vi "WriteReadDrag_YCC.vi"() -> ()   [LabVIEW 2014]
uses:
  (Global) Current handle and LaserPower_YCC.vi
panel:
  in  "Move to Position":bool
  in  "Clear one          all":bool
  in  "Clear Save Position":bool
  in  "Save Position":bool
  in  "Tab Control":enum32{"StandBy", "Drag", "Single WriteRead"}(tab)
  in  "Update new ADC(read) rate":bool
  out "Save Position (um)":dbl[][](array[numeric])
  in  "Clear index (row)":i32
  in  "Move index (row)":i32
  in  "Tab Control":T1(tab)
  in  "ADC Rate for 20bit (ms)":T2(ring)
  out "Sampling Rate for reading (Hz)":dbl
  in  "DAC rate (ms)":dbl=5.0
  out "DAC rate (Hz)":dbl
  out "XY Position":cluster{"X":dbl, "Y":dbl}[](graph)
  in  "Z  (um)":dbl=50.0 format="%.4f"
  out "Current Z (um)":dbl
  in  "Move Z?":bool
  in  "Adjust to Single Read":bool
  in  "Chang X?":bool
  in  "X Move to (um)":dbl=50.0 format="%_6g"
  in  "Chang Y?":bool
  in  "Y Move to (um)":dbl=50.0 format="%_6g"
  in  "Z Move to (um)":dbl=50.0 format="%_6g"
  in  "Chang Z?":bool
  in  "milliseconds to wait":u32=200
  out "Current Position Z (um)":dbl format="%.4f"
  out "Current Position Y (um)":dbl format="%.4f"
  out "Current Position X (um)":dbl format="%.4f"
  in  "read #":i32=1
  in  "Adjust to cursor":bool=TRUE
  in  "Move to (50,50,50) ?":bool
  in  "STOP":bool
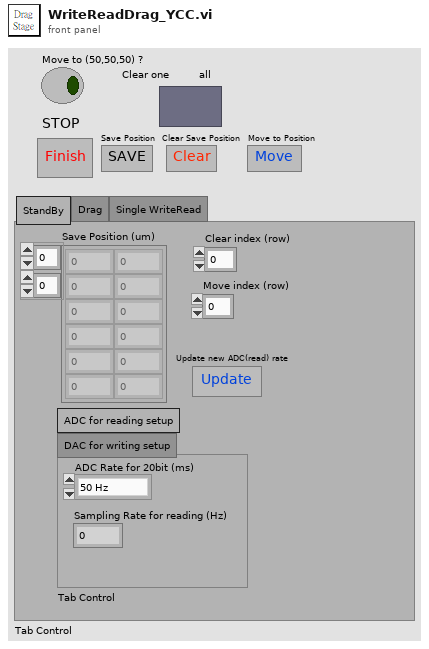
[diagram p1: front panel]
types:
  T1 = enum32{"ADC for reading setup", "DAC for writing setup"}
  T2 = enum16{"50 Hz", "60 Hz", "100 Hz", "500 Hz", "1000 Hz", "2000 Hz", "3750 Hz"}
  T3 = enum16{"StandBy", "Drag", "Single WriteRead", "Move to 50,50,50"}
  T4 = cluster{"Real Current Commanded position (um)":dbl, "Real Current Commanded position (um)":dbl}
  T5 = typedef "LVPointDoubleTypeDef.ctl" = cluster{"Cursor X":dbl, "Cursor Y":dbl}
  T6 = cluster{"position (um)":dbl, "position (um)":dbl}
  T7 = cluster{"Position wrote to three axis (um)":dbl, "Position wrote to three axis (um)":dbl}
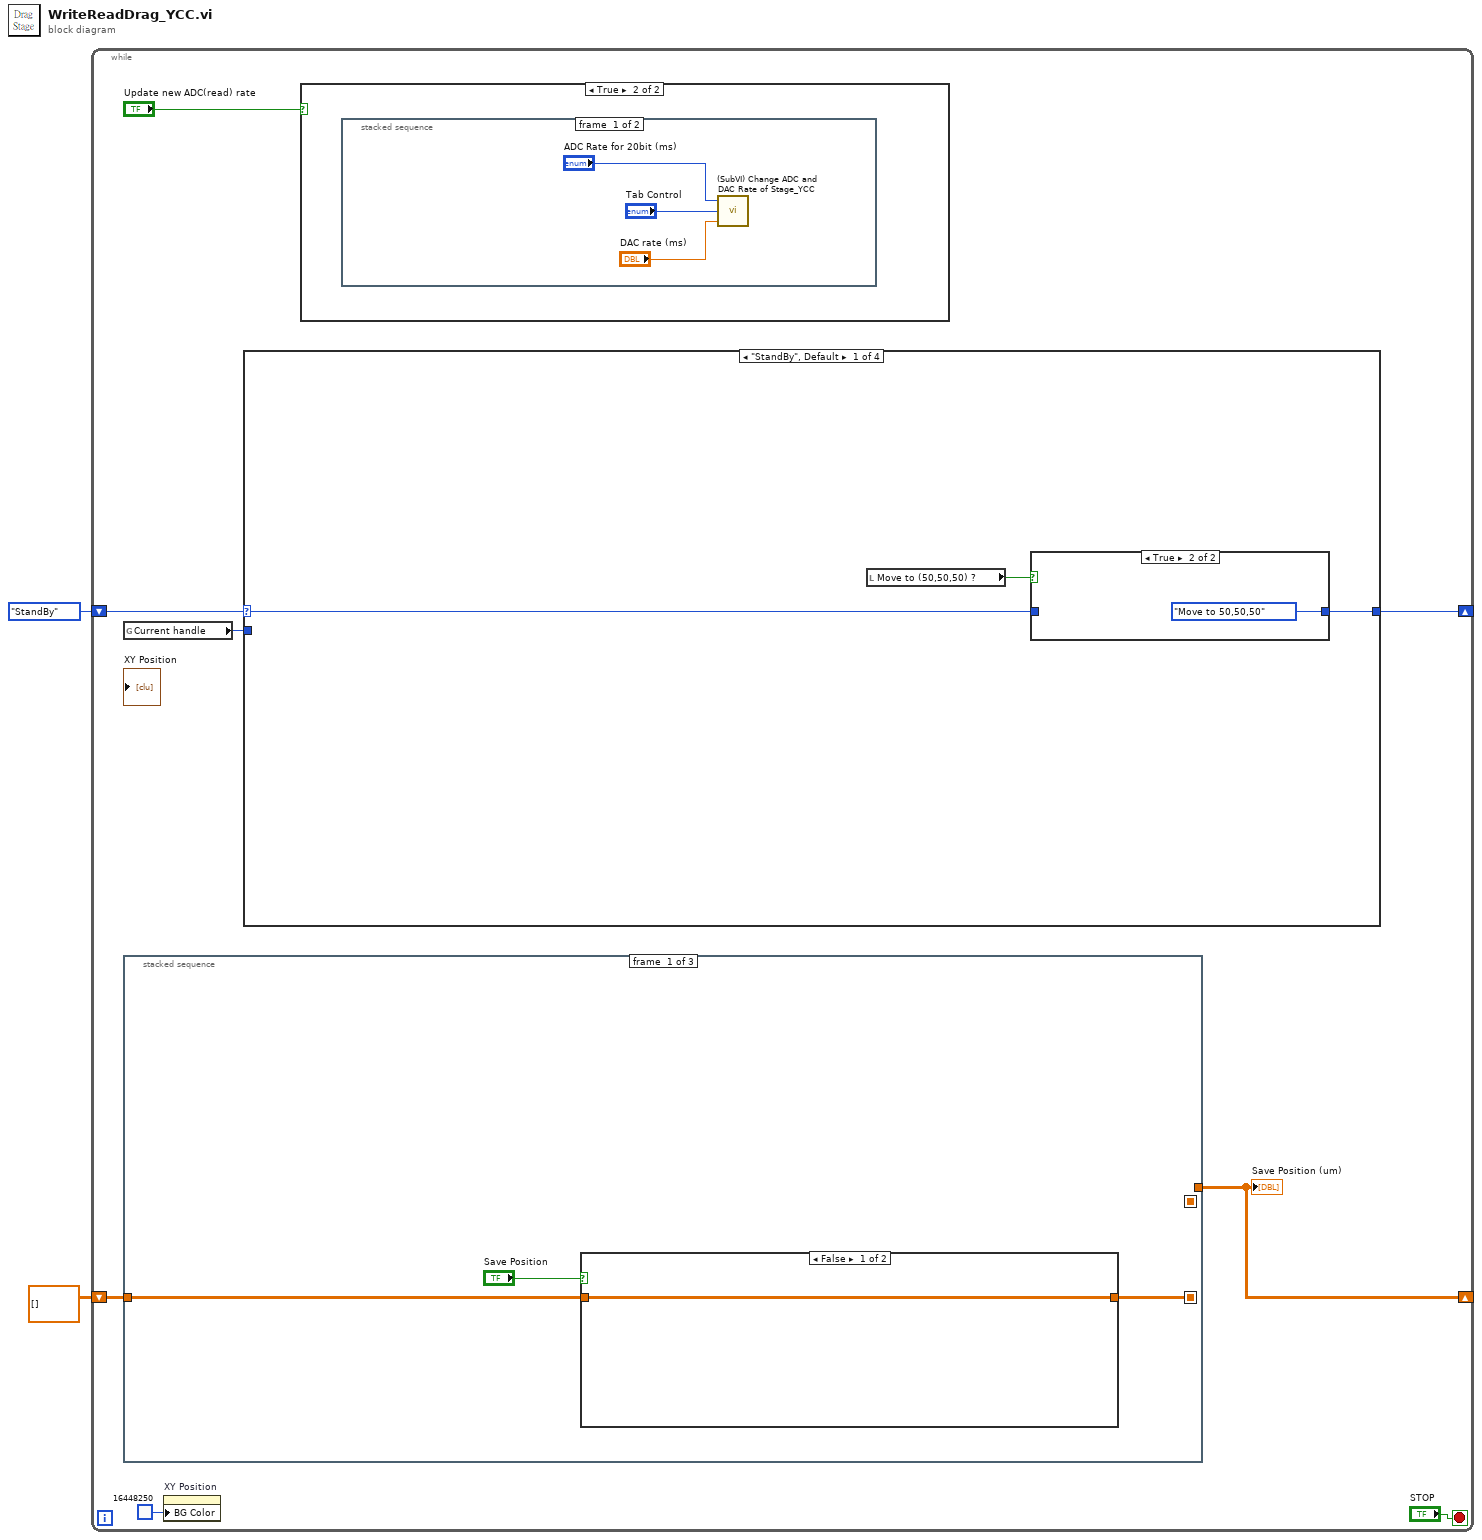
[diagram p0: block diagram]
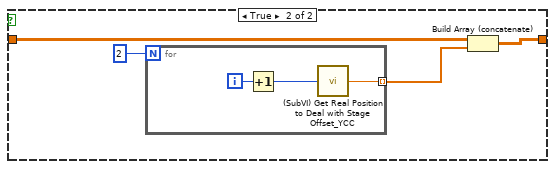
[diagram p2: hidden frame]
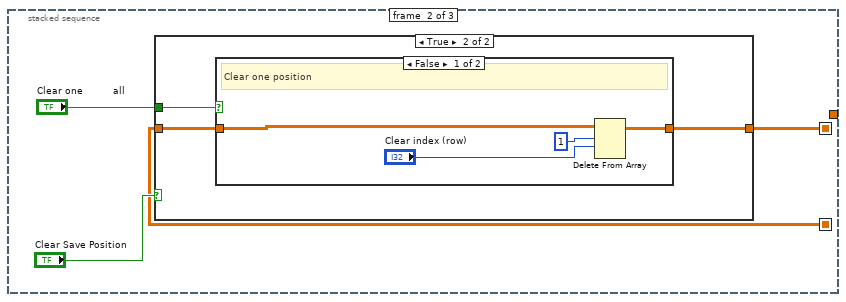
[diagram p3: hidden frame]
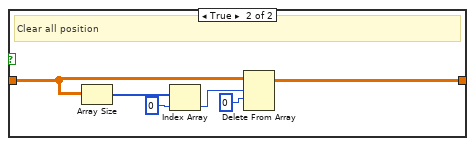
[diagram p5: hidden frame]
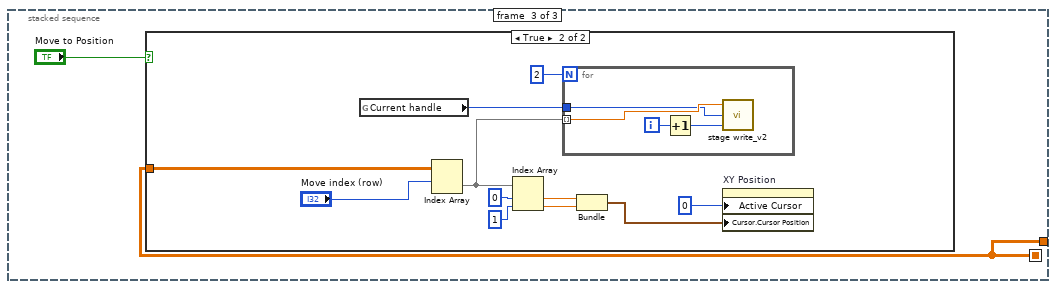
[diagram p6: hidden frame]
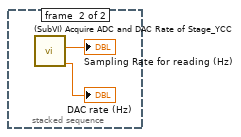
[diagram p9: hidden frame]
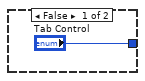
[diagram p10: hidden frame]
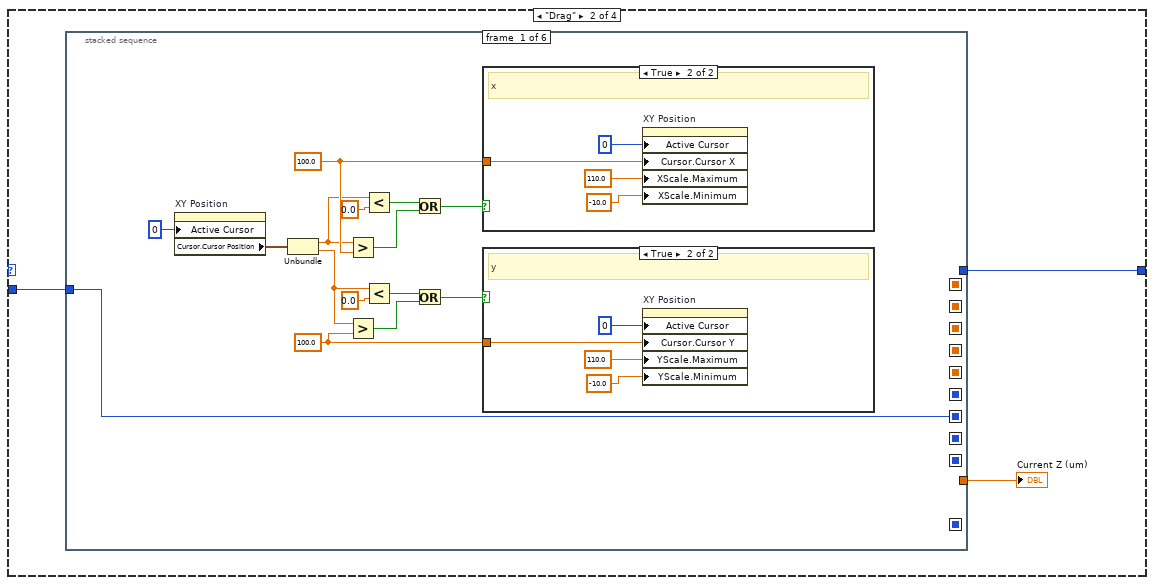
[diagram p11: hidden frame]
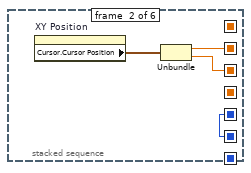
[diagram p14: hidden frame]
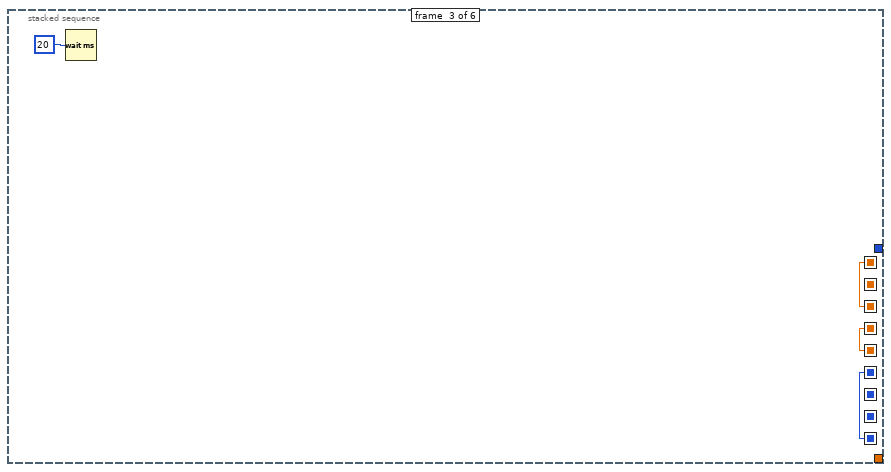
[diagram p15: hidden frame]
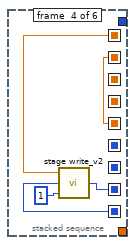
[diagram p16: hidden frame]
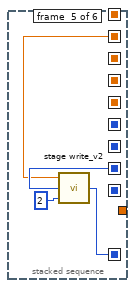
[diagram p17: hidden frame]
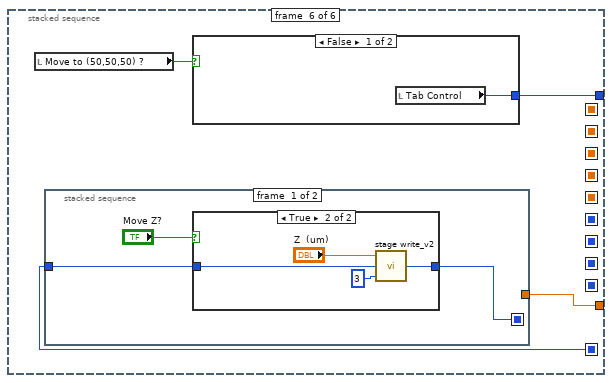
[diagram p18: hidden frame]
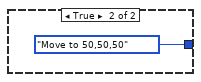
[diagram p19: hidden frame]
diagram:
  n1 = while {
    shift-right: [w10] -> _
    shift-left: T3."StandBy" ("Enum") -> [w8]
    shift-right: [w5] -> _
    shift-left: dbl[][] [] -> [w6]
    stop <- "STOP" stop-if-true
    n2 = global read "(Global) Current handle and LaserPower_YCC.vi" "Current handle"() -> (w7:i32)
    n3 = stacked-sequence {
      seq-local: [w11 _ _] -> [_ w23 _]
      seq-local: [_ w24 _] -> [_ _ w41]
      tunnel: w6 -> [w12 _ _]
      tunnel: [_ _ w41] -> w5
      frame #0 {
        n4 = case shown="False" "Save Position" {
          tunnel: [w14 w16] -> w11
          tunnel: w12 -> [w14 w15]
          frame False {
          }
          frame True {
            n5 = for {
              N: 2 -> [_]
              tunnel: [w19] -> w17 mode=indexing
              i -> [w21]
              n6 = Increment(x=w21) -> (x+1=w20:i32)
              n7 = call "(SubVI) Get Real Position to Deal with Stage Offset_YCC.vi"("Axis"=w20) -> ("Real Current Commanded position (um)"=w19:dbl)  [unwired: 3 in, 1 out]
            }
            n8 = Build Array (concatenate)(w15, w17) -> (w16:dbl[][])
          }
        }
      }
      frame #1 {
        n9 = case shown="True" "Clear Save Position" {
          tunnel: [w26 w27] -> w24
          tunnel: w23 -> [w26 w28]
          tunnel: "Clear one          all" -> [_ w29]
          frame False {
          }
          frame True {
            n10 = case shown="False" w29 {
              tunnel: w28 -> [w33 w39]
              tunnel: [w31 w34] -> w27
              frame False {
                # "Clear one position"
                n11 = Delete From Array(array=w33, length=1, index (row)="Clear index (row)") -> (array with subset deleted=w31:dbl[][])  [unwired: 1 in, 1 out]
              }
              frame True {
                # "Clear all position"
                n12 = Array Size(array=w39) -> (size(s)=w38:i32[])
                n13 = Index Array(array=w38, index=0) -> (element=w36:i32)
                n14 = Delete From Array(array=w39, length=w36, index (row)=0) -> (array with subset deleted=w34:dbl[][])  [unwired: 1 in, 1 out]
              }
            }
          }
        }
      }
      frame #2 {
        n15 = case shown="True" "Move to Position" {
          tunnel: w41 -> [_ w52]
          frame False {
          }
          frame True {
            n16 = global read "(Global) Current handle and LaserPower_YCC.vi" "Current handle"() -> (w49:i32)
            n17 = Index Array(array=w52, index (row)="Move index (row)") -> (element=w47:dbl[])  [unwired: 1 in]
            n18 = Index Array(array=w47, index #1=0 ("index"), index #2=1 ("index")) -> (element #1=w44:dbl, element #2=w43:dbl)
            n19 = for {
              N: 2 -> [_]
              tunnel: w47 -> [w56] mode=indexing
              tunnel: w49 -> [w53]
              i -> [w55]
              n20 = Increment(x=w55) -> (x+1=w54:i32)
              n21 = call "stage write_v2.vi"("axis"=w54, "Incoming Handle"=w53, "position"=w56) -> ()  [unwired: 2 in, 1 out]
            }
            n22 = Bundle("Real Current Commanded position (um)"=w44, "Real Current Commanded position (um)"=w43) -> (w42:T4)  [unwired: 1 in]
            n23 = property on="XY Position" class="XYGraph (strict)"("Active Cursor"=u32 0, "Cursor.Cursor Position"=w42) -> ()  [unwired: 2 in, 2 out]
          }
        }
      }
    }
    "Save Position (um)" <- w5
    n24 = property on="XY Position" class="XYGraph (strict)"("BG Color"=u32 16448250) -> ()  [unwired: 2 in, 2 out]
    n25 = case shown="\"StandBy\", Default" w8 {
      selector: w8 -> [w62 _ _ _]
      tunnel: [w63 w67 w128 w190] -> w10
      tunnel: w7 -> [_ w69 w129 w189]
      frame "StandBy", Default {
        n26 = local read "Move to (50,50,50) ?"() -> (w64:bool)
        n27 = case shown="True" w64 {
          tunnel: ["Tab Control" T3."Move to 50,50,50" ("Enum")] -> w63
          tunnel: w62 -> [_ _]
          frame False {
          }
          frame True {
          }
        }
      }
      frame "Drag" {
        n28 = stacked-sequence {
          seq-local: [w70 _ _ _ _ _] -> [_ w93 _ _ _ _]
          seq-local: [_ w93 _ _ _ _] -> [_ _ w99 _ _ _]
          seq-local: [_ w94 _ _ _ _] -> [_ _ w98 _ _ _]
          seq-local: [_ w95 _ _ _ _] -> [_ _ w97 _ _ _]
          seq-local: [_ _ w99 _ _ _] -> [_ _ _ w105 _ _]
          seq-local: [_ _ w98 _ _ _] -> [_ _ _ w101 _ _]
          seq-local: [_ _ w97 _ _ _] -> [_ _ _ w102 _ _]
          seq-local: [_ _ _ w101 _ _] -> [_ _ _ _ w107 _]
          seq-local: [_ _ _ w103 _ _] -> [_ _ _ _ w108 _]
          seq-local: [_ _ _ _ w106 _] -> [_ _ _ _ _ w113]
          tunnel: w69 -> [w70 _ _ _ _ _]
          tunnel: [_ _ _ _ _ w112] -> w68
          tunnel: [_ _ _ _ _ w110] -> w67
          frame #0 {
            w82 = 100.0 ("y")
            w83 = 100.0 ("y")
            n29 = property on="XY Position" class="XYGraph (strict)"("Active Cursor"=u32 0) -> ("Cursor.Cursor Position"=w84:T5)  [unwired: 2 in, 2 out]
            n30 = Unbundle(w84) -> ("Cursor X"=w80:dbl, "Cursor Y"=w77:dbl)
            n31 = Greater?(x=w80, y=w83) -> (0:w75:bool)
            n32 = Greater?(x=w77, y=w82) -> (0:w72:bool)
            n33 = Less?(x=w80, y=0.0) -> (x < y?=w76:bool)
            n34 = Less?(x=w77, y=0.0) -> (x < y?=w73:bool)
            n35 = Or(x=w76, y=w75) -> (x .or. y?=w74:bool)
            n36 = Or(x=w73, y=w72) -> (x .or. y?=w71:bool)
            n37 = case shown="True" w74 {
              tunnel: w83 -> [_ w92]
              frame False {
              }
              frame True {
                # "x"
                n38 = property on="XY Position" class="XYGraph (strict)"("Active Cursor"=u32 0, "Cursor.Cursor X"=w92, "XScale.Maximum"=110.0 ("X Scale.Range:Maximum"), "XScale.Minimum"=-10.0 ("X Scale.Range:Minimum")) -> ()  [unwired: 2 in, 2 out]
              }
            }
            n39 = case shown="True" w71 {
              tunnel: w82 -> [_ w88]
              frame False {
              }
              frame True {
                # "y"
                n40 = property on="XY Position" class="XYGraph (strict)"("Active Cursor"=u32 0, "Cursor.Cursor Y"=w88, "YScale.Maximum"=110.0 ("X Scale.Range:Maximum"), "YScale.Minimum"=-10.0 ("X Scale.Range:Minimum")) -> ()  [unwired: 2 in, 2 out]
              }
            }
          }
          frame #1 {
            n41 = property on="XY Position" class="XYGraph (strict)"() -> ("Cursor.Cursor Position"=w96:T5)  [unwired: 2 in, 2 out]
            n42 = Unbundle(w96) -> ("Cursor X"=w95:dbl, "Cursor Y"=w94:dbl)
          }
          frame #2 {
            n43 = Wait (ms)(milliseconds to wait=u32 20) -> ()  [unwired: 1 out]
          }
          frame #3 {
            n44 = call "stage write_v2.vi"("axis"=u32 1, "Incoming Handle"=w105, "position"=w102) -> ("out handle"=w103:i32)  [unwired: 2 in]
          }
          frame #4 {
            n45 = call "stage write_v2.vi"("axis"=u32 2, "Incoming Handle"=w108, "position"=w107) -> ("out handle"=w106:i32)  [unwired: 2 in]
          }
          frame #5 {
            n46 = local read "Move to (50,50,50) ?"() -> (w111:bool)
            n47 = stacked-sequence {
              seq-local: [w116 _] -> [_ w126]
              tunnel: w113 -> [w118 _]
              tunnel: [_ w124] -> w112
              frame #0 {
                n48 = case shown="True" "Move Z?" {
                  tunnel: w118 -> [w119 w122]
                  tunnel: [w119 w120] -> w116
                  frame False {
                  }
                  frame True {
                    n49 = call "stage write_v2.vi"("axis"=u32 3, "Incoming Handle"=w122, "position"="Z  (um)") -> ("out handle"=w120:i32)  [unwired: 2 in]
                  }
                }
              }
              frame #1 {
                n50 = call "stage read_v2.vi"("Axis"=u32 3 ("axis"), "Incoming Handle"=w126, "read #"=1) -> ("position (um)"=w124:dbl)  [unwired: 1 in, 1 out]
              }
            }
            n51 = case shown="False" w111 {
              tunnel: [w114 T3."Move to 50,50,50" ("Enum")] -> w110
              frame False {
                n52 = local read "Tab Control"() -> (w114:enum32{"StandBy", "Drag", "Single WriteRead"})
              }
              frame True {
              }
            }
          }
        }
        "Current Z (um)" <- w68
      }
      frame "Single WriteRead" {
        n53 = stacked-sequence {
          seq-local: [w130 _ _ _ _ _ _ _] -> [_ w138 _ _ _ _ _ _]
          seq-local: [_ w138 _ _ _ _ _ _] -> [_ _ w143 _ _ _ _ _]
          seq-local: [_ _ w143 _ _ _ _ _] -> [_ _ _ w148 _ _ _ _]
          seq-local: [_ _ _ w148 _ _ _ _] -> [_ _ _ _ w152 _ _ _]
          seq-local: [_ _ _ _ w151 _ _ _] -> [_ _ _ _ _ w167 _ _]
          seq-local: [_ _ _ _ w150 _ _ _] -> [_ _ _ _ _ w166 _ _]
          seq-local: [_ _ _ _ _ w167 _ _] -> [_ _ _ _ _ _ w171 _]
          seq-local: [_ _ _ _ _ w166 _ _] -> [_ _ _ _ _ _ w170 _]
          tunnel: w129 -> [w131 _ _ _ _ _ _ _]
          tunnel: [_ _ _ _ _ w164 _ _] -> w128
          frame #0 {
            # "write x"
            n54 = case shown="False" "Chang X?" {
              tunnel: w131 -> [w133 w135]
              tunnel: [w133 w134] -> w130
              frame False {
              }
              frame True {
                n55 = call "stage write_v2.vi"("axis"=u32 1, "Incoming Handle"=w135, "position"="X Move to (um)") -> ("out handle"=w134:i32)  [unwired: 2 in]
              }
            }
          }
          frame #1 {
            # "write y"
            n56 = case shown="True" "Chang Y?" {
              tunnel: w138 -> [_ w140]
              frame False {
              }
              frame True {
                n57 = call "stage write_v2.vi"("axis"=u32 2, "Incoming Handle"=w140, "position"="Y Move to (um)") -> ()  [unwired: 2 in, 1 out]
              }
            }
          }
          frame #2 {
            n58 = case shown="True" "Chang Z?" {
              tunnel: w143 -> [_ w145]
              frame False {
              }
              frame True {
                n59 = call "stage write_v2.vi"("axis"=u32 3, "Incoming Handle"=w145, "position"="Z Move to (um)") -> ()  [unwired: 2 in, 1 out]
              }
            }
          }
          frame #3 {
            n60 = Wait (ms)(milliseconds to wait="milliseconds to wait") -> ()  [unwired: 1 out]
          }
          frame #4 {
            n61 = for {
              N: 3 -> [_]
              tunnel: [w160] -> w157 mode=indexing
              tunnel: w152 -> [w159]
              i -> [w163]
              n62 = Increment(x=w163) -> (x+1=w162:i32)
              n63 = call "stage read_v2.vi"("Axis"=w162, "Incoming Handle"=w159, "read #"="read #") -> ("position (um)"=w160:dbl)  [unwired: 1 in, 1 out]
            }
            n64 = Index Array(array=w157, index #1=0 ("index"), index #2=1 ("index"), index #3=2 ("index")) -> (element #1=w151:dbl, element #2=w150:dbl, element #3=→"Current Position Z (um)":dbl)
            "Current Position X (um)" <- w151
            "Current Position Y (um)" <- w150
          }
          frame #5 {
            n65 = local read "Move to (50,50,50) ?"() -> (w165:bool)
            n66 = case shown="False" w165 {
              tunnel: [w168 T3."Move to 50,50,50" ("Enum")] -> w164
              frame False {
                n67 = local read "Tab Control"() -> (w168:enum32{"StandBy", "Drag", "Single WriteRead"})
              }
              frame True {
              }
            }
          }
          frame #6 {
            n68 = case shown="True" "Adjust to cursor" {
              tunnel: w171 -> [_ w174]
              tunnel: w170 -> [_ w173]
              frame False {
              }
              frame True {
                n69 = Bundle("position (um)"=w174, "position (um)"=w173) -> (w175:T6)  [unwired: 1 in]
                n70 = property on="XY Position" class="XYGraph (strict)"("Cursor.Cursor Position"=w175) -> ()  [unwired: 2 in, 2 out]
              }
            }
          }
          frame #7 {
            n71 = case shown="True" "Adjust to Single Read" {
              frame False {
              }
              frame True {
                n72 = stacked-sequence {
                  seq-local: [w177 _] -> [_ w188]
                  frame #0 {
                    n73 = for {
                      N: 3 -> [_]
                      tunnel: [w179] -> w177 mode=indexing
                      i -> [w181]
                      n74 = Increment(x=w181) -> (x+1=w180:i32)
                      n75 = call "(SubVI) Get Real Position to Deal with Stage Offset_YCC.vi"("Axis"=w180) -> ("Real Current Commanded position (um)"=w179:dbl)  [unwired: 3 in, 1 out]
                    }
                  }
                  frame #1 {
                    n76 = Index Array(array=w188, index #1=0 ("index"), index #2=1 ("index"), index #3=2 ("index")) -> (element #1=w184:dbl, element #2=w183:dbl, element #3=w182:dbl)
                    n77 = local write "X Move to (um)"(w184) -> ()
                    n78 = local write "Y Move to (um)"(w183) -> ()
                    n79 = local write "Z Move to (um)"(w182) -> ()
                  }
                }
              }
            }
          }
        }
      }
      frame "Move to 50,50,50" {
        w190 = T3."StandBy" ("Enum")
        n80 = case shown="True" "Move to (50,50,50) ?" {
          tunnel: w189 -> [_ w192]
          frame False {
          }
          frame True {
            n81 = stacked-sequence {
              seq-local: [w193 _] -> [_ w195]
              tunnel: w192 -> [w194 _]
              frame #0 {
                w193 = 50.0 ("Position wrote to three axis (um)")
                n82 = call "(SubVI) Write to Three Axises_YCC.vi"("handle"=w194, "Position wrote to three axis (um)"=w193) -> ()  [unwired: 3 in]
              }
              frame #1 {
                n83 = Bundle("Position wrote to three axis (um)"=w195, "Position wrote to three axis (um)"=w195) -> (w196:T7)  [unwired: 1 in]
                n84 = property on="XY Position" class="XYGraph (strict)"("Cursor.Cursor Position"=w196) -> ()  [unwired: 2 in, 2 out]
              }
            }
          }
        }
        n85 = local write "Tab Control"(w190) -> ()
      }
    }
    n86 = case shown="True" "Update new ADC(read) rate" {
      frame False {
      }
      frame True {
        n87 = stacked-sequence {
          frame #0 {
            n88 = call "(SubVI) Change ADC and DAC Rate of Stage_YCC.vi"("ADC Rate for 20bit (ms)"="ADC Rate for 20bit (ms)", "Tab Control"="Tab Control", "DAC rate (ms)"="DAC rate (ms)") -> ()  [unwired: 2 in, 2 out]
          }
          frame #1 {
            n89 = call "(SubVI) Acquire ADC and DAC Rate of Stage_YCC.vi"() -> ("adcfreq-read (Hz)"=→"Sampling Rate for reading (Hz)":dbl, "dacfreq-write (Hz)"=→"DAC rate (Hz)":dbl)  [unwired: 2 in, 2 out]
          }
        }
      }
    }
  }
